vi "RemoveGroup Value Change.vi"(11 "References":T1) -> (0 "error out":errorcluster)   [LabVIEW 2015, in "TDMS datalogger editor node.lvclass"]
uses:
  TDMS datalogger editor node.lvclass
  <vilib>/NI/DCAF/Tag Editor Core/Table API/Table Manager/object ref.ctl
  <vilib>/NI/DCAF/Tag Editor Core/Configuration Editor/Classes/Engine Parent/Engine Parent Editor Node.lvclass
  <vilib>/NI/DCAF/Tag Editor Core/Configuration Editor/Classes/Module editor node/module editor node.lvclass
  TDMS datalogger editor node.lvclass/TDMS datalogger editor node.ctl
  <vilib>/NI/DCAF/Tag Editor Core/Table API/Table Manager/Table Manager.lvclass
panel:
  in  "Groups":string(tree)="group1"
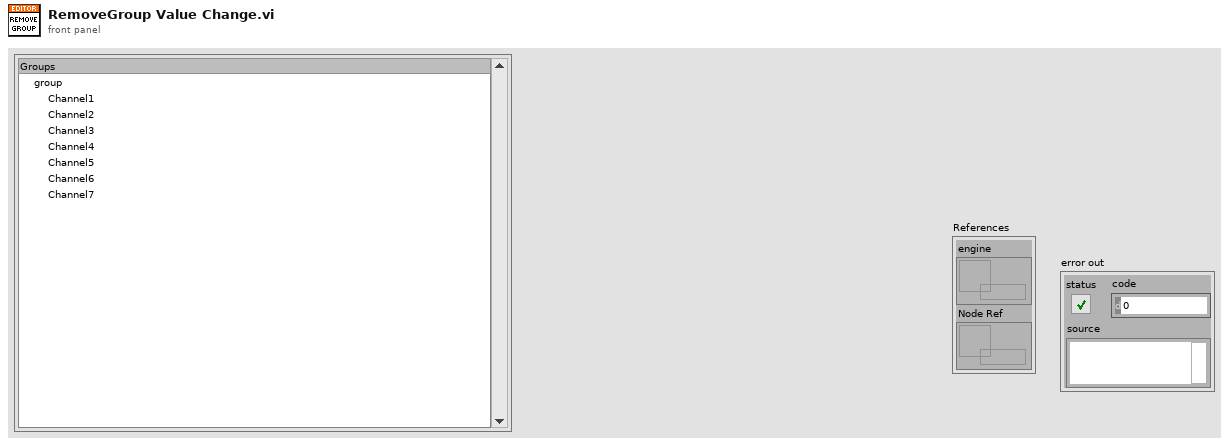
[diagram p1: front panel]
types:
  T1 = typedef "Table Manager.lvlib/Table Manager.lvclass/object ref.ctl" = cluster{"engine":refnum<data-value>, "Node Ref":refnum<data-value>}
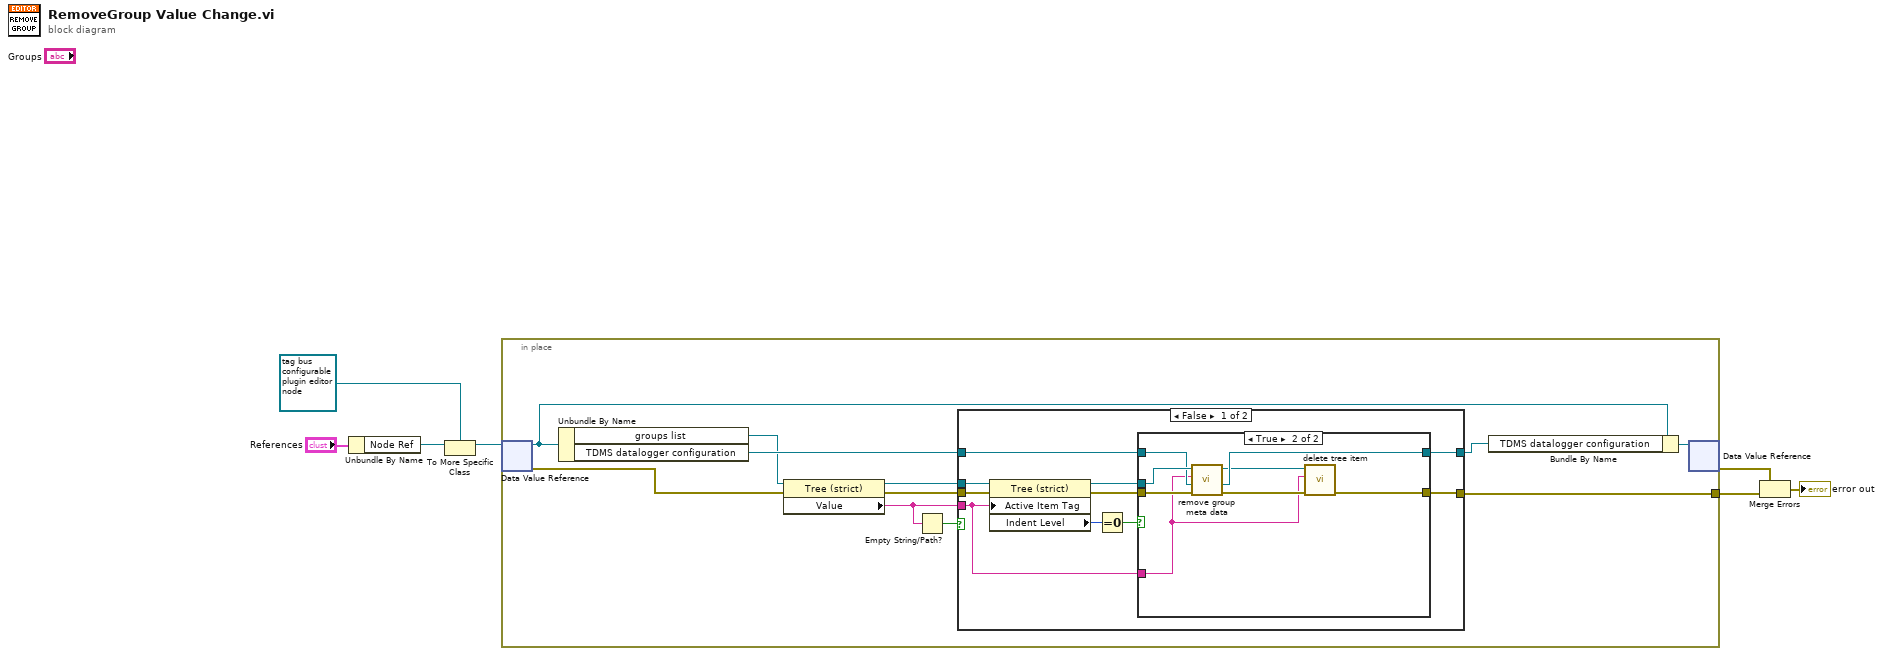
[diagram p0: block diagram]
diagram:
  n1 = Unbundle By Name("References") -> ("Node Ref"=w4:refnum<data-value>)
  n2 = To More Specific Class(target class=refnum<data-value> refnum ("data value reference"), reference=w4) -> (specific class reference=w2:refnum<data-value>)  [unwired: 1 in, 1 out]
  n3 = in-place {
    in-place-border: [w16] -> w7
    n4 = in-place-dvr #1(w2) -> (w14:refnum<class "TDMS datalogger editor node.lvclass">, w11:errorcluster)
    n5 = Unbundle By Name(w14) -> ("groups list"=w10:refnum<vi>, "TDMS datalogger configuration"=w17:refnum<class "TDMS datalogger configuration.lvclass">)
    n6 = property class="Tree (strict)"(reference=w10, error in=w11) -> (reference out=w9:refnum<vi>, "Value"=w8:string)  [unwired: 1 out]
    n7 = Empty String/Path?(string/path=w8) -> (empty?=w15:bool)
    n8 = case shown="False" w15 {
      tunnel: w9 -> [w23 _]
      tunnel: w11 -> [w22 w39]
      tunnel: w17 -> [w21 w38]
      tunnel: [w20 w39] -> w16
      tunnel: w8 -> [w19 _]
      tunnel: [w18 w38] -> w12
      frame False {
        n9 = property class="Tree (strict)"(reference=w23, error in=w22, "Active Item Tag"=w19) -> (reference out=w27:refnum<vi>, error out=w26:errorcluster, "Indent Level"=w25:i32)
        n10 = Equal To 0?(x=w25) -> (x = 0?=w24:bool)
        n11 = case shown="True" w24 {
          tunnel: [w29 w30] -> w20
          tunnel: w27 -> [_ w37]
          tunnel: w19 -> [_ w32]
          tunnel: w26 -> [w29 w35]
          tunnel: w21 -> [w28 w36]
          tunnel: [w28 w34] -> w18
          frame False {
            # "Do nothing on channel items"
          }
          frame True {
            n12 = call "remove group meta data.vi"("error in (no error)"=w35, "TDMS datalogger configuration in"=w36, "group tag"=w32, "tree reference"=w37) -> ("error out"=w33:errorcluster, "TDMS datalogger configuration out"=w34:refnum<class "TDMS datalogger configuration.lvclass">, "tree reference out"=w31:refnum<vi>)  [unwired: 5 in]
            n13 = call "delete tree item.vi"("error in"=w33, "Tag"=w32, "tree reference in"=w31) -> ("error out"=w30:errorcluster)  [unwired: 7 in, 1 out]
          }
        }
      }
      frame True {
      }
    }
    n14 = Bundle By Name(cluster=w14, "TDMS datalogger configuration"=w12) -> (w13:refnum<class "TDMS datalogger editor node.lvclass">)
    n15 = in-place-dvr #1(w13) -> (w6:errorcluster)  [unwired: 1 out]
  }
  n16 = Merge Errors(w6, w7) -> (→"error out":errorcluster)
